vi "Main Page.vi"(8 "error in (no error)":errorcluster, 11 "Node Ptr":T2 format="%.0x") -> (0 "error out":errorcluster)   [LabVIEW 2015, in "J1939 Addon System Explorer.lvlib"]
uses:
  J1939 Addon System Explorer.lvlib
  <vilib>/NI Veristand/Custom Device API/Custom Device Item Ref.ctl
  Types/XNET Port.ctl
  Shared/Types/XNET Settings.ctl
  <vilib>/NI Veristand/Custom Device API/Custom Device File Dependency.ctl
  <vilib>/NI Veristand/Custom Device API/Path Specification.ctl
  <vilib>/NI Veristand/Custom Device API/Path Type.ctl
  <vilib>/NI Veristand/Custom Device API/Custom Device Supported Target.ctl
  Shared/SubVIs/Constants.vi
  <vilib>/NI Veristand/Custom Device API/Get Item Property (Boolean).vi
  <vilib>/NI Veristand/Custom Device API/Get Item Property (Variant).vi
  <vilib>/NI Veristand/Custom Device API/Set Item Property (Boolean).vi
  <vilib>/NI Veristand/Custom Device API/Set Item Property (U16).vi
  <vilib>/NI Veristand/Custom Device API/Set Item Property (Path).vi
  <vilib>/NI Veristand/Custom Device API/Get Item Property (U16).vi
  <vilib>/NI Veristand/Custom Device API/Get Item Property (Path).vi
  <vilib>/NI Veristand/Custom Device API/Set Item Property (Variant).vi
  <vilib>/NI VeriStand/Custom Device API/Custom Device API.lvlib
  Shared/J1939 Addon Shared.lvlib
panel:
  in  "Write Decimation":u32=1
  in  "Outcoming Process Rate [Hz]":u32=100
  in  "Incoming Process Rate [Hz]":u32=100
  in  "J1939 Settings 3":cluster{"Section Name":string}={"Section Name"="NI 986x Settings"}
  in  "J1939 Database Settings":cluster{"Section Name":string}={"Section Name"="J1939 Database Settings"}
  in  "RIO Device":u16
  in  "Bitfile Path":path
  in  "Enable Bitfile":bool
  in  "Termination":enum16{"Off", "On"}(ring)
  in  "SHDocVw.IWebBrowser2":refnum<k7>(container)
  in  "NI 986x Settings":cluster{"Section Name":string}={"Section Name"="J1939 Settings"}
  in  "XNET CAN Port":T1 items=["CAN 1", "CAN 2", "CAN 3", "CAN 4", "CAN 5", "CAN 6", "CAN 7", "CAN 8"]
  in  "Baud rate [Bd]":u32 format="%.0p"
  out "XNET Cluster":refnum<k21>
  out "XNET Database":refnum<k21>
  in  "Name":string
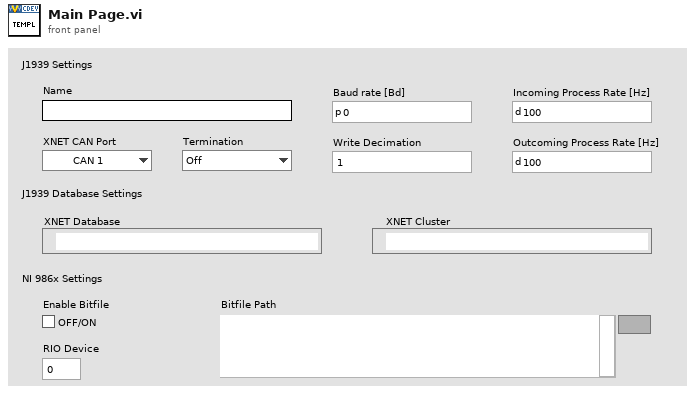
[diagram p1: front panel]
types:
  T1 = typedef "J1939 Addon System Explorer.lvlib/XNET Port.ctl" = u16
  T2 = typedef "Custom Device API.lvlib/Custom Device Item Ref.ctl" = u64
  T3 = typedef "J1939 Addon Shared.lvlib/XNET Settings.ctl" = cluster{"Database":refnum<k21>, "Cluster":refnum<k21>, "Port":string, "Baud rate [Bd]":u32, "Termination":u32, "Incoming Rate":u32, "Outcoming Rate":u32, "Write Decimation":u32}
  T4 = typedef "Custom Device API.lvlib/Custom Device Item Info.ctl" = cluster{"Name":string, "Is Channel":bool, "GUID":string, "Is Waveform":bool}
  T5 = typedef "Custom Device API.lvlib/Custom Device File Dependency.ctl" = cluster{"Source":T6, "RT Destination":path, "ForceDownload?":bool, "SupportedTarget":T8, "Version":string}
  T6 = typedef "Custom Device API.lvlib/Path Specification.ctl" = cluster{"Path":path, "Type":T7}
  T7 = typedef "Custom Device API.lvlib/Path Type.ctl" = enum16{"Absolute", "To Base", "To Common Data Dir", "To Application Data Dir"}
  T8 = typedef "Custom Device API.lvlib/Custom Device Supported Target.ctl" = enum16{"All", "PharLap", "VxWorks", "Windows", "Linux_32_ARM", "Linux_x64", "PharLap & Windows", "PharLap & VxWorks", "VxWorks & Windows"}
  T9 = typedef "Custom Device API.lvlib/Custom Device Commands.ctl" = enum16{"Default", "Item renamed", "Shutdown", "Dynamic button pressed"}
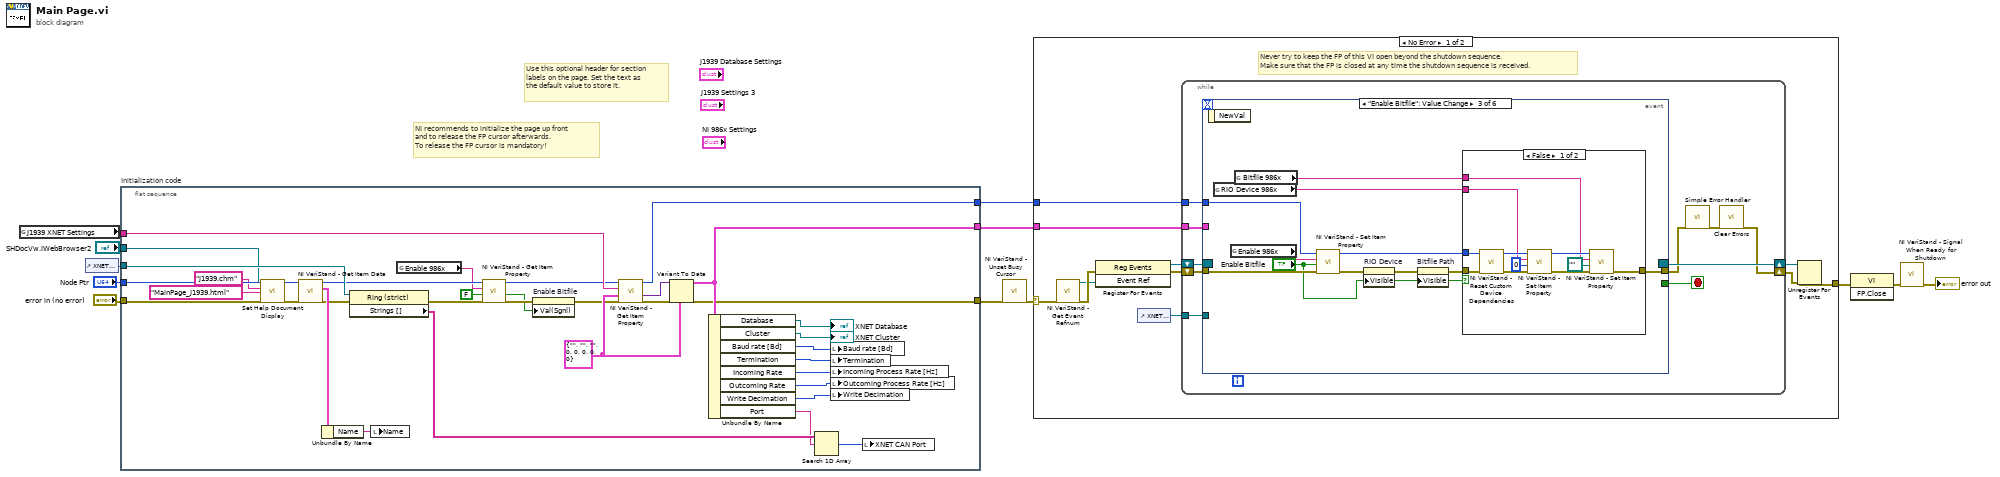
[diagram p0: block diagram]
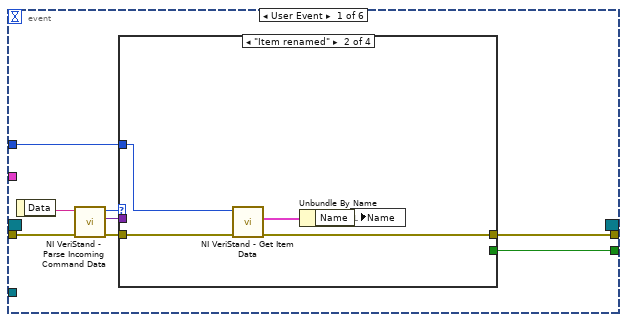
[diagram p2: hidden frame]
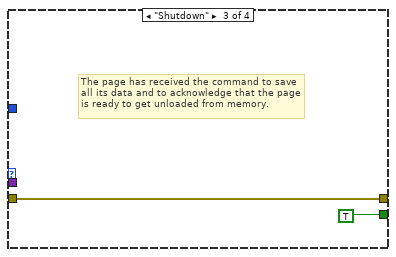
[diagram p4: hidden frame]
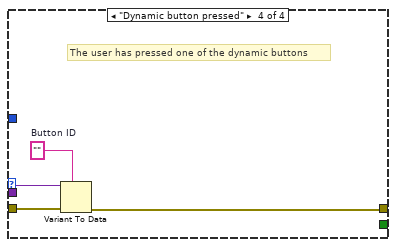
[diagram p5: hidden frame]
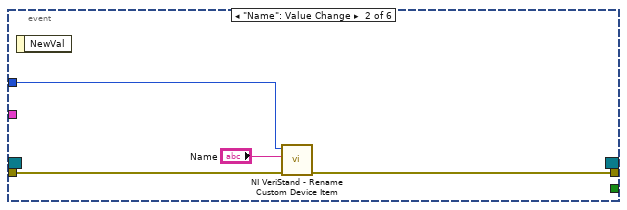
[diagram p6: hidden frame]
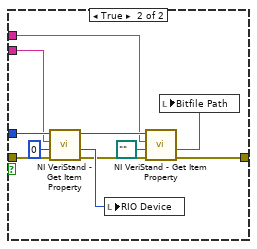
[diagram p7: hidden frame]
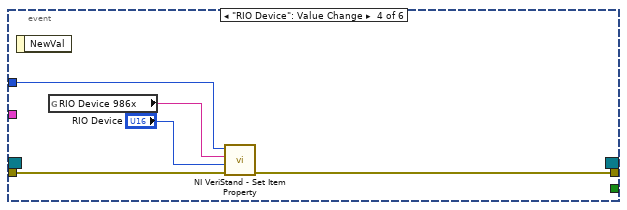
[diagram p8: hidden frame]
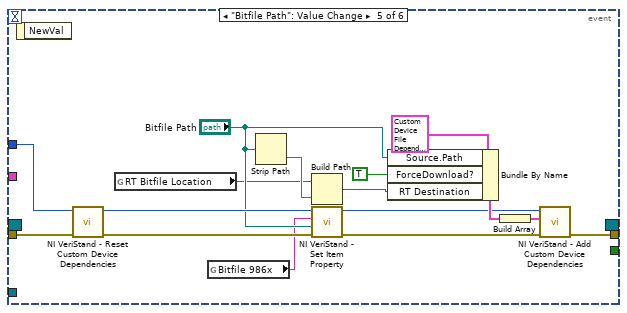
[diagram p9: hidden frame]
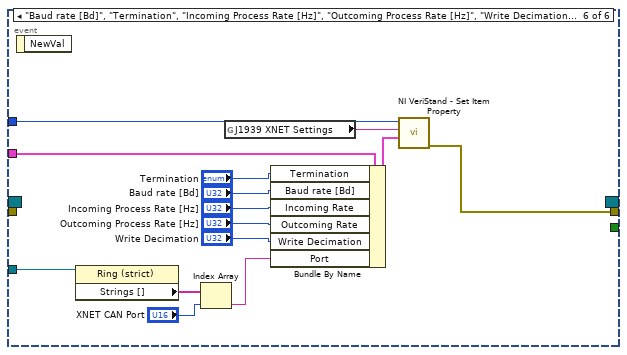
[diagram p10: hidden frame]
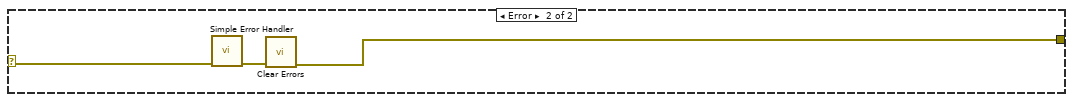
[diagram p11: hidden frame]
diagram:
  # "Use this optional header for section labels on the page. Set the text as the default value to store it."
  # "NI recommends to initialize the page up front\nand to release the FP cursor afterwards.\nTo release the FP cursor is mandatory!"
  n1 = global read "Constants.vi" "J1939 XNET Settings"() -> (w3:string)
  n2 = control-ref of="XNET CAN Port"() -> (w4:refnum<vi>)
  n3 = flat-sequence "Initialization code" {
    tunnel: "error in (no error)" -> [w30]
    tunnel: "Node Ptr" -> [w34]
    tunnel: [w15] -> w8
    tunnel: [w45] -> w5
    tunnel: w4 -> [w36]
    tunnel: w3 -> [w35]
    tunnel: "SHDocVw.IWebBrowser2" -> [w31]
    tunnel: [w26] -> w1
    frame #0 {
      w42 = T3 {"Database"="", "Cluster"="", "Port"="", "Baud rate [Bd]"=0, "Termination"=0, "Incoming Rate"=0, "Outcoming Rate"=0, "Write Decimation"=0} ("J1939 XNET Settings")
      n4 = call "Set Help Document Display.vi"("error in (no error)"=w30, "HTML File"="MainPage_J1939.html", "Main CHM File"="J1939.chm", "SHDocVw.IWebBrowser2"=w31) -> ("error out"=w29:errorcluster)  [unwired: 7 in]
      n5 = call <vilib>:"NI VeriStand - Get Item Data.vi"("error in (no error)"=w29, "Item Ref in"=w34) -> ("error out"=w37:errorcluster, "Item Info"=w47:T4, "Item Ref out"=w24:T2)  [unwired: 7 out]
      n6 = Unbundle By Name(w47) -> ("Name"=w46:string)
      n7 = property class="Ring (strict)"(reference=w36, error in=w37) -> (error out=w25:errorcluster, "Strings []"=w40:string[])  [unwired: 1 out]
      n8 = local write "Name"(w46) -> ()
      n9 = global read "Constants.vi" "Enable 986x"() -> (w22:string)
      n10 = call-poly <vilib>:"NI VeriStand - Get Item Property.vi"("error in (no error)"=w25, "Default Value"=FALSE, "Property Name"=w22, "Item Ref in"=w24) -> ("error out"=w21:errorcluster, "Value"=w19:bool, "Item Ref out"=w23:T2)  [unwired: 4 in, 1 out]
      n11 = property on="Enable Bitfile" class="Bool (strict)"(error in=w21, "Val(Sgnl)"=w19) -> (error out=w20:errorcluster)  [unwired: 1 in, 1 out]
      n12 = call-poly <vilib>:"NI VeriStand - Get Item Property.vi"("error in (no error)"=w20, "Default Value"=w42, "Property Name"=w35, "Item Ref in"=w23) -> ("error out"=w44:errorcluster, "Value"=w43:variant, "Item Ref out"=w45:T2)  [unwired: 4 in, 1 out]
      n13 = Variant To Data(error in=w44, type=w42, Variant=w43) -> (data=w26:T3, error out=w15:errorcluster)
      n14 = Unbundle By Name(w26) -> ("Database"=→"XNET Database":refnum<k21>, "Cluster"=→"XNET Cluster":refnum<k21>, "Baud rate [Bd]"=w41:u32, "Termination"=w16:u32, "Incoming Rate"=w17:u32, "Outcoming Rate"=w18:u32, "Write Decimation"=w13:u32, "Port"=w39:string)
      n15 = Search 1D Array(1D array=w40, element=w39) -> (index of element=w38:i32)  [unwired: 1 in]
      n16 = local write "Baud rate [Bd]"(w41) -> ()
      n17 = local write "Termination"(w16) -> ()
      n18 = local write "Incoming Process Rate [Hz]"(w17) -> ()
      n19 = local write "Outcoming Process Rate [Hz]"(w18) -> ()
      n20 = local write "Write Decimation"(w13) -> ()
      n21 = local write "XNET CAN Port"(w38) -> ()
    }
  }
  n22 = call <vilib>:"NI VeriStand - Unset Busy Cursor.vi"("error in (no error)"=w8) -> ("error out"=w7:errorcluster)  [unwired: 10 out]
  n23 = case shown="No Error" w7 {
    selector: w7 -> [w50 w163]
    tunnel: [w55 w161] -> w12
    tunnel: w5 -> [w51 _]
    tunnel: w1 -> [w49 _]
    frame No Error {
      # "Never try to keep the FP of this VI open beyond the shutdown sequence.\nMake sure that the FP is closed at any time the shutdown sequence is received."
      n24 = call <vilib>:"NI VeriStand - Get Event Refnum.vi"("error in (no error)"=w50) -> ("error out"=w58:errorcluster, "Event Ref"=w54:refnum<user-event>)  [unwired: 9 out]
      n25 = register-events(error in=w58, w54) -> (reference out=w52:refnum<event-registration>, error out=w53:errorcluster)  [unwired: 1 in]
      n26 = control-ref of="XNET CAN Port"() -> (w48:refnum<vi>)
      n27 = while {
        tunnel: w51 -> [w64]
        shift-right: [w61] -> w56
        shift-left: w53 -> [w67]
        shift-right: [w68] -> w57
        shift-left: w52 -> [w66]
        tunnel: w49 -> [w60]
        tunnel: w48 -> [w59]
        stop <- w65 stop-if-true
        n28 = event shown="[2] \"Enable Bitfile\": Value Change" {
          selector: w66 -> [_ _ _ _ _ _]
          dyn-events: [_ _ _ _ _ _] -> w68
          timeout: _ -> [_ _ _ _ _ _]
          tunnel: w67 -> [w76 w92 w103 w130 w146 _]
          tunnel: [w72 _ _ _ _ _] -> w65
          tunnel: [w71 w91 w96 w129 w144 w155] -> w63
          tunnel: w64 -> [w70 w90 w102 w128 w145 w153]
          tunnel: w60 -> [_ _ _ _ _ w154]
          tunnel: w59 -> [_ _ _ _ _ w157]
          event User Event {
            n29 = event-data() -> ("Data"=w75:string)  [unwired: 1 out]
            n30 = call <vilib>:"NI VeriStand - Parse Incoming Command Data.vi"("error in (no error)"=w76, "Incoming data"=w75) -> ("error out"=w74:errorcluster, "Outgoing data"=w69:variant, "Action"=w73:T9)  [unwired: 7 out]
            n31 = case shown="\"Item renamed\"" w73 {
              tunnel: w74 -> [w77 w82 w83 w88]
              tunnel: [_ _ TRUE _] -> w72
              tunnel: [w77 w79 w83 w85] -> w71
              tunnel: w70 -> [_ w81 _ _]
              tunnel: w69 -> [_ _ _ w87]
              frame "Default", Default {
              }
              frame "Item renamed" {
                n32 = call <vilib>:"NI VeriStand - Get Item Data.vi"("error in (no error)"=w82, "Item Ref in"=w81) -> ("error out"=w79:errorcluster, "Item Info"=w80:T4)  [unwired: 8 out]
                n33 = Unbundle By Name(w80) -> ("Name"=w78:string)
                n34 = local write "Name"(w78) -> ()
              }
              frame "Shutdown" {
                # "The page has received the command to save all its data and to acknowledge that the page is ready to get unloaded from memory."
              }
              frame "Dynamic button pressed" {
                w86 = ""  # Button ID
                # "The user has pressed one of the dynamic buttons"
                n35 = Variant To Data(error in=w88, type=w86, Variant=w87) -> (error out=w85:errorcluster)  [unwired: 1 out]
              }
            }
          }
          event "Name": Value Change {
            n36 = event-data() -> ()  [unwired: 2 out]
            n37 = call <vilib>:"NI VeriStand - Rename Custom Device Item.vi"("error in (no error)"=w92, "New Name"="Name", "Item Ref in"=w90) -> ("error out"=w91:errorcluster)  [unwired: 1 in, 7 out]
          }
          event "Enable Bitfile": Value Change {
            n38 = event-data() -> ()  [unwired: 2 out]
            n39 = global read "Constants.vi" "RIO Device 986x"() -> (w94:string)
            n40 = global read "Constants.vi" "Enable 986x"() -> (w101:string)
            n41 = global read "Constants.vi" "Bitfile 986x"() -> (w93:string)
            n42 = call-poly <vilib>:"NI VeriStand - Set Item Property.vi"("error in (no error)"=w103, "Value"="Enable Bitfile", "Property Name"=w101, "Item Ref in"=w102) -> ("error out"=w99:errorcluster, "Item Ref out"=w95:T2)  [unwired: 5 in, 1 out]
            n43 = property on="RIO Device" class="DigNum (strict)"(error in=w99, "Visible"="Enable Bitfile") -> (error out=w100:errorcluster)  [unwired: 1 in, 1 out]
            n44 = property on="Bitfile Path" class="Path"(error in=w100, "Visible"="Enable Bitfile") -> (error out=w97:errorcluster)  [unwired: 1 in, 1 out]
            n45 = case shown="False" "Enable Bitfile" {
              tunnel: w97 -> [w114 w125]
              tunnel: [w110 w119] -> w96
              tunnel: w95 -> [w113 w124]
              tunnel: w94 -> [w107 w123]
              tunnel: w93 -> [w106 w116]
              frame False {
                n46 = call <vilib>:"NI VeriStand - Reset Custom Device Dependencies.vi"("error in (no error)"=w114, "Device Ref in"=w113) -> ("error out"=w111:errorcluster, "Device Ref out"=w109:T2)  [unwired: 8 in]
                n47 = call-poly <vilib>:"NI VeriStand - Set Item Property.vi"("error in (no error)"=w111, "Value"=u16 0, "Property Name"=w107, "Item Ref in"=w109) -> ("error out"=w112:errorcluster, "Item Ref out"=w108:T2)  [unwired: 5 in, 1 out]
                n48 = call-poly <vilib>:"NI VeriStand - Set Item Property.vi"("error in (no error)"=w112, "Value"=path "", "Property Name"=w106, "Item Ref in"=w108) -> ("error out"=w110:errorcluster)  [unwired: 5 in, 2 out]
              }
              frame True {
                n49 = call-poly <vilib>:"NI VeriStand - Get Item Property.vi"("error in (no error)"=w125, "Default Value"=u16 0, "Property Name"=w123, "Item Ref in"=w124) -> ("error out"=w120:errorcluster, "Value"=w121:u16, "Item Ref out"=w117:T2)  [unwired: 4 in, 1 out]
                n50 = local write "RIO Device"(w121) -> ()
                n51 = call-poly <vilib>:"NI VeriStand - Get Item Property.vi"("error in (no error)"=w120, "Default Value"=path "", "Property Name"=w116, "Item Ref in"=w117) -> ("error out"=w119:errorcluster, "Value"=w115:path)  [unwired: 4 in, 2 out]
                n52 = local write "Bitfile Path"(w115) -> ()
              }
            }
          }
          event "RIO Device": Value Change {
            n53 = event-data() -> ()  [unwired: 2 out]
            n54 = global read "Constants.vi" "RIO Device 986x"() -> (w127:string)
            n55 = call-poly <vilib>:"NI VeriStand - Set Item Property.vi"("error in (no error)"=w130, "Value"="RIO Device", "Property Name"=w127, "Item Ref in"=w128) -> ("error out"=w129:errorcluster)  [unwired: 5 in, 2 out]
          }
          event "Bitfile Path": Value Change {
            n56 = event-data() -> ()  [unwired: 2 out]
            n57 = call <vilib>:"NI VeriStand - Reset Custom Device Dependencies.vi"("error in (no error)"=w146, "Device Ref in"=w145) -> ("error out"=w137:errorcluster, "Device Ref out"=w134:T2)  [unwired: 8 in]
            n58 = global read "Constants.vi" "RT Bitfile Location"() -> (w131:path)
            n59 = global read "Constants.vi" "Bitfile 986x"() -> (w132:string)
            n60 = Strip Path(path="Bitfile Path") -> (name=w139:string)  [unwired: 1 out]
            n61 = Build Path(base path=w131, name or relative path=w139) -> (appended path=w138:path)
            n62 = call-poly <vilib>:"NI VeriStand - Set Item Property.vi"("error in (no error)"=w137, "Value"="Bitfile Path", "Property Name"=w132, "Item Ref in"=w134) -> ("error out"=w136:errorcluster, "Item Ref out"=w135:T2)  [unwired: 5 in, 1 out]
            n63 = Bundle By Name(cluster=T5 {"Source"={"Path"=path "", "Type"=enum."Absolute"}, "RT Destination"=path "", "ForceDownload?"=FALSE, "SupportedTarget"=enum."PharLap", "Version"=""} ("Dependency"), "Source.Path"="Bitfile Path", "ForceDownload?"=TRUE, "RT Destination"=w138) -> (w142:T5)
            n64 = Build Array(w142) -> (w141:T5[])
            n65 = call <vilib>:"NI VeriStand - Add Custom Device Dependencies.vi"("error in (no error)"=w136, "Dependencies"=w141, "Device Ref in"=w135) -> ("error out"=w144:errorcluster)  [unwired: 7 in, 1 out]
          }
          event "Baud rate [Bd]", "Termination", "Incoming Process Rate [Hz]", "Outcoming Process Rate [Hz]", "Write Decimation": Value Change {
            n66 = event-data() -> ()  [unwired: 2 out]
            n67 = property on="Property Node" class="Ring (strict)"(reference=w157) -> ("Strings []"=w160:string[])  [unwired: 1 in, 2 out]
            n68 = Index Array(array=w160, index="XNET CAN Port") -> (element=w151:string)
            n69 = global read "Constants.vi" "J1939 XNET Settings"() -> (w156:string)
            n70 = Bundle By Name(cluster=w154, "Termination"="Termination", "Baud rate [Bd]"="Baud rate [Bd]", "Incoming Rate"="Incoming Process Rate [Hz]", "Outcoming Rate"="Outcoming Process Rate [Hz]", "Write Decimation"="Write Decimation", "Port"=w151) -> (w152:T3)
            n71 = call-poly <vilib>:"NI VeriStand - Set Item Property.vi"("Value"=w152, "Property Name"=w156, "Item Ref in"=w153) -> ("error out"=w155:errorcluster)  [unwired: 6 in, 2 out]
          }
        }
        n72 = call <vilib>:"Simple Error Handler.vi"("error in (no error)"=w63) -> ("error out"=w62:errorcluster)  [unwired: 1 in, 7 out]
        n73 = call <vilib>:"Clear Errors.vi"("error in (no error)"=w62) -> ("error out"=w61:errorcluster)  [unwired: 1 in, 5 out]
      }
      n74 = Unregister For Events(event registration refnum=w57, error in=w56) -> (error out=w55:errorcluster)
    }
    frame Error {
      n75 = call <vilib>:"Simple Error Handler.vi"("error in (no error)"=w163) -> ("error out"=w162:errorcluster)  [unwired: 1 in, 7 out]
      n76 = call <vilib>:"Clear Errors.vi"("error in (no error)"=w162) -> ("error out"=w161:errorcluster)  [unwired: 1 in, 5 out]
    }
  }
  n77 = invoke class="VI" method="FP.Close"(error in=w12) -> (error out=w11:errorcluster)  [unwired: 2 in, 2 out]
  n78 = call <vilib>:"NI VeriStand - Signal When Ready for Shutdown.vi"("error in (no error)"=w11) -> ("error out"=→"error out":errorcluster)  [unwired: 10 out]
